vi "SequenceRunner.vi"() -> ()   [LabVIEW 2019]
uses:
  Components/B_Globals.vi
  Components/Global 2.vi
  Components/DeltaRamp_globals.vi
panel:
  in  "B_rate":dbl
  in  "T_rate":dbl
  out "Output File":path
  in  "Directory":path
  in  "T_high":dbl
  in  "T_low":dbl
  in  "Skip":bool
  out "Step":dbl
  out "Of":dbl
  out "Action":string="Waiting for go"
  in  "Start":bool
  in  "Array":T1(array[cluster])
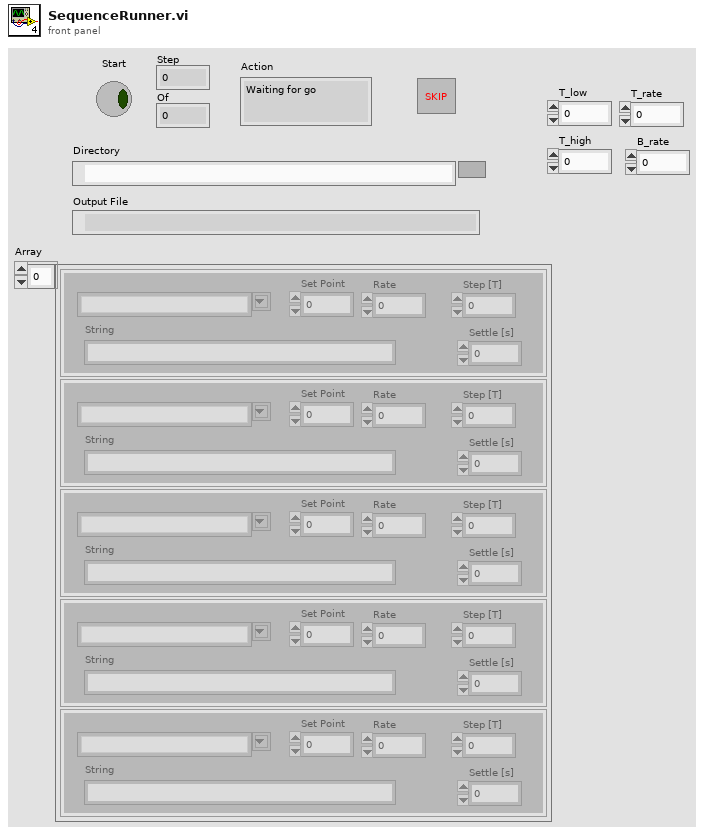
[diagram p1: front panel]
types:
  T1 = cluster{"Combo Box":string, "Rate":dbl, "Set Point":dbl, "String":string, "Step [T]":dbl, "Settle [s]":dbl}[]
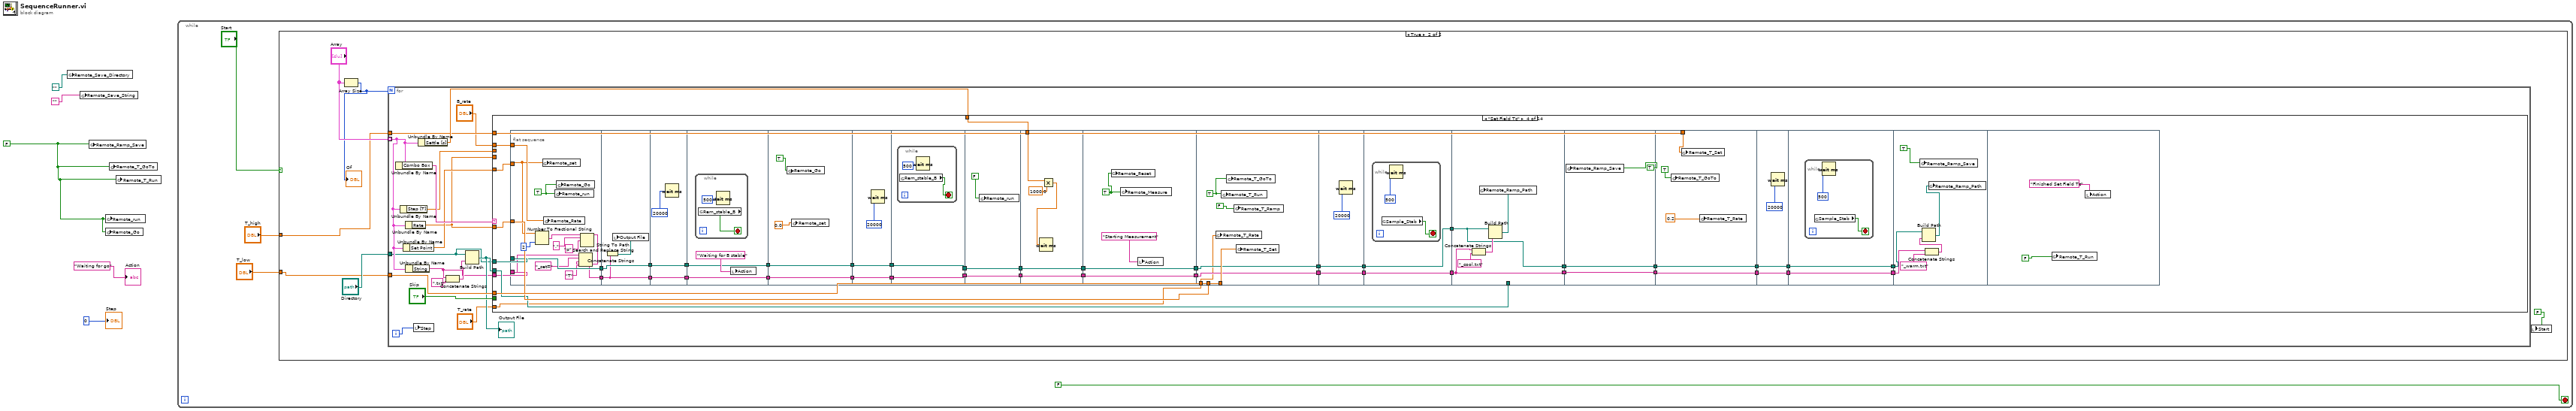
[diagram p0: block diagram]
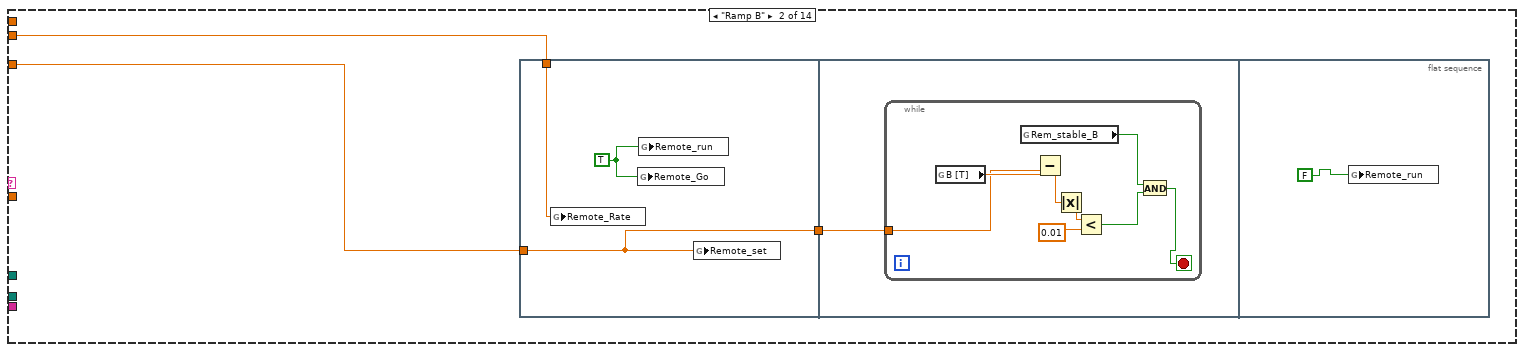
[diagram p4: hidden frame]
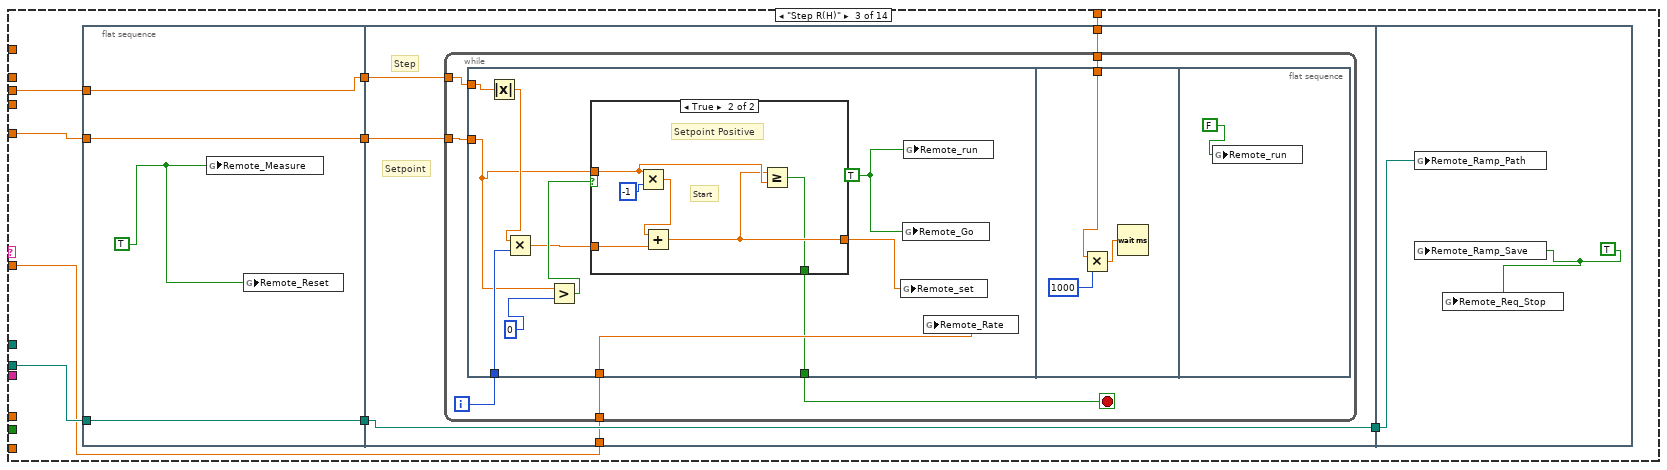
[diagram p5: hidden frame]
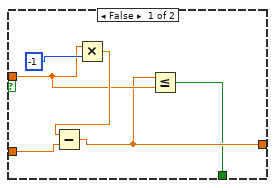
[diagram p6: hidden frame]
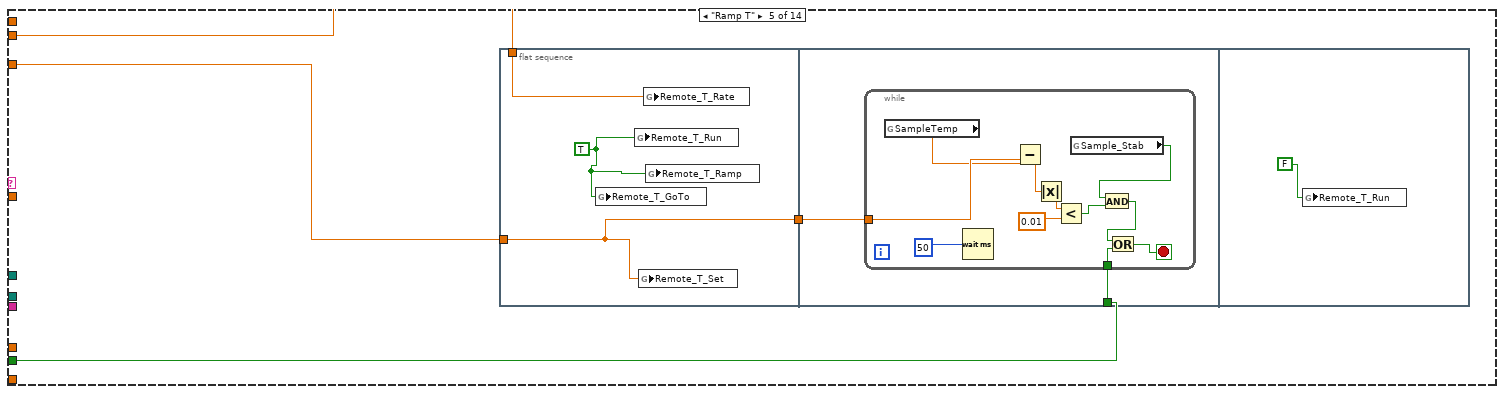
[diagram p7: hidden frame]
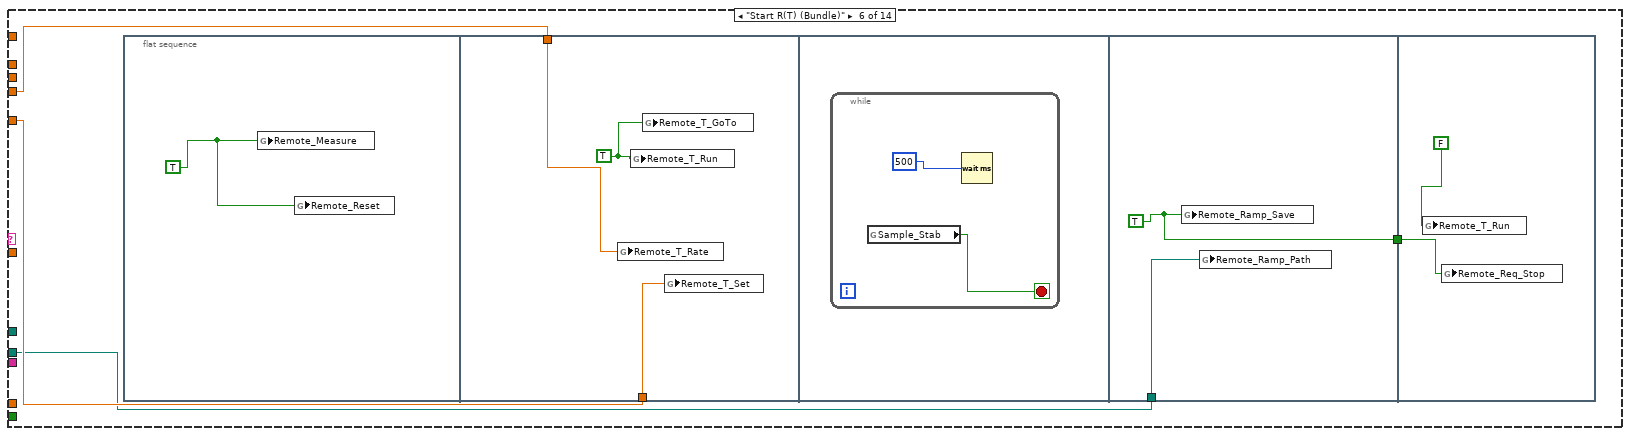
[diagram p8: hidden frame]
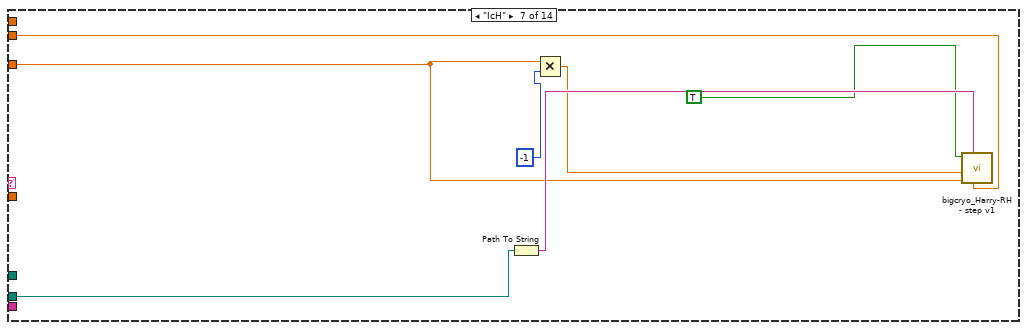
[diagram p9: hidden frame]
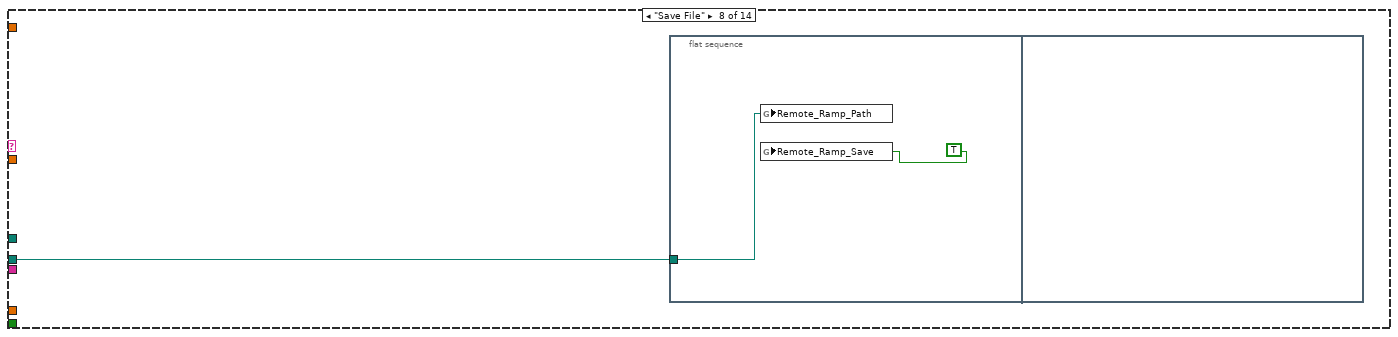
[diagram p10: hidden frame]
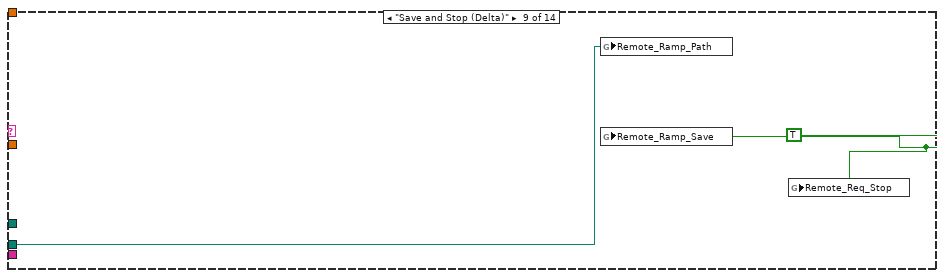
[diagram p11: hidden frame]
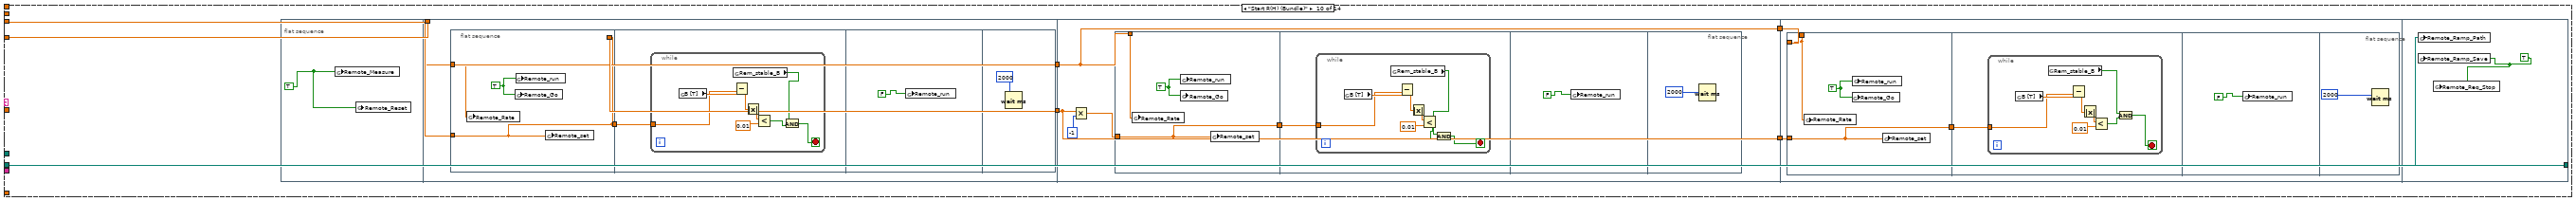
[diagram p12: hidden frame]
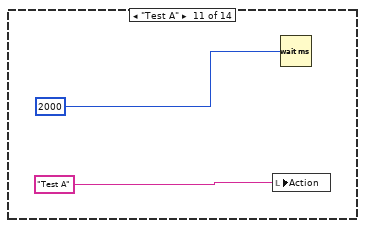
[diagram p13: hidden frame]
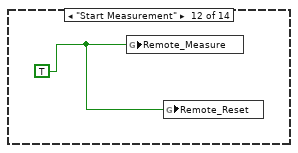
[diagram p14: hidden frame]
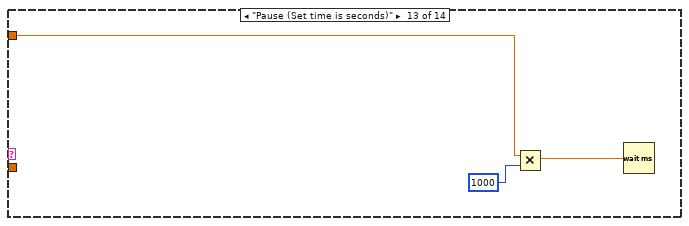
[diagram p15: hidden frame]
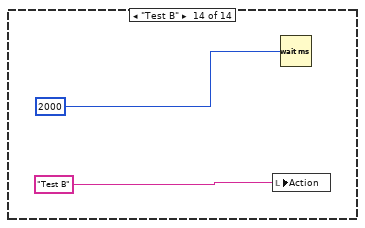
[diagram p16: hidden frame]
diagram:
  w5 = FALSE
  n1 = global write "DeltaRamp_globals.vi" "Remote_Save_Directory"(path "") -> ()
  n2 = global write "DeltaRamp_globals.vi" "Remote_Save_String"("") -> ()
  n3 = global write "DeltaRamp_globals.vi" "Remote_Ramp_Save"(w5) -> ()
  n4 = global write "B_Globals.vi" "Remote_Go"(w5) -> ()
  n5 = global write "B_Globals.vi" "Remote_run"(w5) -> ()
  n6 = global write "Global 2.vi" "Remote_T_GoTo"(w5) -> ()
  n7 = global write "Global 2.vi" "Remote_T_Run"(w5) -> ()
  n8 = while {
    stop <- FALSE stop-if-true
    n9 = case shown="True" "Start" {
      tunnel: "T_high" -> [_ w10]
      tunnel: "T_low" -> [_ w11]
      frame False {
      }
      frame True {
        n10 = Array Size(array="Array") -> (size(s)=w13:i32)
        "Of" <- w13
        n11 = for {
          N: w13 -> [_]
          tunnel: "Array" -> [w28] mode=indexing
          tunnel: "Directory" -> [w18]
          tunnel: w11 -> [w22]
          tunnel: w10 -> [w21]
          i -> [w30]
          n12 = Unbundle By Name(w28) -> ("Combo Box"=w32:string)
          n13 = Unbundle By Name(w28) -> ("Step [T]"=w26:dbl)
          n14 = Unbundle By Name(w28) -> ("Set Point"=w31:dbl)
          n15 = Unbundle By Name(w28) -> ("Rate"=w25:dbl)
          n16 = Unbundle By Name(w28) -> ("String"=w19:string)
          n17 = local write "Step"(w30) -> ()
          n18 = Unbundle By Name(w28) -> ("Settle [s]"=w27:dbl)
          n19 = Concatenate Strings(w19, ".txt") -> (w23:string)
          n20 = Build Path(base path=w18, name or relative path=w23) -> (appended path=w20:path)
          "Output File" <- w20
          n21 = case shown="\"Set Field Tc\"" w32 {
            tunnel: w31 -> [_ w35 w53 w147 w237 w260 w272 _ _ w289 _ _ w351 _]
            tunnel: w25 -> [_ w34 _ _ w238 w259 w277 _ _ w288 _ _ _ _]
            tunnel: w20 -> [_ _ w56 w142 _ w258 w274 w278 w282 w283 _ _ _ _]
            tunnel: "Skip" -> [_ _ _ _ w236 _ _ _ _ _ _ _ _ _]
            tunnel: w27 -> [_ _ w51 w146 _ _ _ _ _ _ _ _ _ _]
            tunnel: w26 -> [_ _ w50 _ _ _ _ _ _ _ _ _ _ _]
            tunnel: w25 -> [_ _ w49 w144 _ _ _ _ _ _ _ _ _ _]
            tunnel: w22 -> [_ _ _ w145 _ _ _ _ _ _ _ _ _ _]
            tunnel: w21 -> [_ _ _ w143 _ _ _ _ _ _ _ _ _ _]
            tunnel: w19 -> [_ _ _ w141 _ _ _ _ _ _ _ _ _ _]
            tunnel: w18 -> [_ _ _ w134 _ _ _ _ _ _ _ _ _ _]
            tunnel: "B_rate" -> [_ _ _ w111 _ _ _ _ _ _ _ _ _ _]
            tunnel: "T_rate" -> [_ _ _ w110 _ _ _ _ _ _ _ _ _ _]
            frame "False", Default {
            }
            frame "Ramp B" {
              n22 = flat-sequence {
                tunnel: w35 -> [w36]
                tunnel: w34 -> [w37]
                tunnel: [w36] -> w33
                tunnel: w33 -> [w39]
                frame #0 {
                  w38 = TRUE
                  n23 = global write "B_Globals.vi" "Remote_Rate"(w37) -> ()
                  n24 = global write "B_Globals.vi" "Remote_Go"(w38) -> ()
                  n25 = global write "B_Globals.vi" "Remote_run"(w38) -> ()
                  n26 = global write "B_Globals.vi" "Remote_set"(w36) -> ()
                }
                frame #1 {
                  n27 = while {
                    tunnel: w39 -> [w46]
                    stop <- w40 stop-if-true
                    n28 = global read "B_Globals.vi" "B [T]"() -> (w47:dbl)
                    n29 = global read "B_Globals.vi" "Rem_stable_B"() -> (w42:bool)
                    n30 = Subtract(x=w47, y=w46) -> (x-y=w45:dbl)
                    n31 = Absolute Value(x=w45) -> (abs(x)=w44:dbl)
                    n32 = Less?(x=w44, y=0.01) -> (x < y?=w41:bool)
                    n33 = And(x=w42, y=w41) -> (x .and. y?=w40:bool)
                  }
                }
                frame #2 {
                  n34 = global write "B_Globals.vi" "Remote_run"(FALSE) -> ()
                }
              }
            }
            frame "Step R(H)" {
              n35 = flat-sequence {
                tunnel: [w60] -> w57
                tunnel: w56 -> [w60]
                tunnel: [w59] -> w54
                tunnel: w53 -> [w59]
                tunnel: [w58] -> w52
                tunnel: w50 -> [w58]
                tunnel: w57 -> [w66]
                tunnel: [w66] -> w55
                tunnel: w54 -> [w65]
                tunnel: w52 -> [w64]
                tunnel: w51 -> [w63]
                tunnel: w49 -> [w62]
                tunnel: w55 -> [w100]
                frame #0 {
                  w61 = TRUE
                  n36 = global write "DeltaRamp_globals.vi" "Remote_Measure"(w61) -> ()
                  n37 = global write "DeltaRamp_globals.vi" "Remote_Reset"(w61) -> ()
                }
                frame #1 {
                  # "Step"
                  # "Setpoint"
                  n38 = while {
                    tunnel: w65 -> [w72]
                    tunnel: w64 -> [w70]
                    tunnel: w63 -> [w69]
                    tunnel: w62 -> [w68]
                    i -> [w71]
                    stop <- w67 stop-if-true
                    n39 = flat-sequence {
                      tunnel: w72 -> [w76]
                      tunnel: w71 -> [w82]
                      tunnel: w70 -> [w80]
                      tunnel: w68 -> [w79]
                      tunnel: [w73] -> w67
                      tunnel: w69 -> [w98]
                      frame #0 {
                        w81 = TRUE
                        n40 = Absolute Value(x=w80) -> (abs(x)=w83:dbl)
                        n41 = Multiply(x=w83, y=w82) -> (x*y=w75:dbl)
                        n42 = Greater?(x=w76, y=0) -> (0:w77:bool)
                        n43 = case shown="True" w77 {
                          tunnel: w76 -> [w86 w92]
                          tunnel: w75 -> [w88 w93]
                          tunnel: [w85 w91] -> w74
                          tunnel: [w84 w90] -> w73
                          frame False {
                            n44 = Multiply(x=w86, y=-1) -> (x*y=w87:dbl)
                            n45 = Subtract(x=w87, y=w88) -> (x-y=w85:dbl)
                            n46 = Less Or Equal?(x=w85, y=w86) -> (x <= y?=w84:bool)
                          }
                          frame True {
                            # "Start"
                            # "Setpoint Positive"
                            n47 = Multiply(x=w92, y=-1) -> (x*y=w94:dbl)
                            n48 = Add(x=w94, y=w93) -> (x+y=w91:dbl)
                            n49 = Greater Or Equal?(x=w91, y=w92) -> (x >= y?=w90:bool)
                          }
                        }
                        n50 = global write "B_Globals.vi" "Remote_set"(w74) -> ()
                        n51 = global write "B_Globals.vi" "Remote_Go"(w81) -> ()
                        n52 = global write "B_Globals.vi" "Remote_run"(w81) -> ()
                        n53 = global write "B_Globals.vi" "Remote_Rate"(w79) -> ()
                      }
                      frame #1 {
                        n54 = Multiply(x=w98, y=1000) -> (x*y=w97:dbl)
                        n55 = Wait (ms)(milliseconds to wait=w97) -> ()  [unwired: 1 out]
                      }
                      frame #2 {
                        n56 = global write "B_Globals.vi" "Remote_run"(FALSE) -> ()
                      }
                    }
                  }
                }
                frame #2 {
                  w101 = TRUE
                  n57 = global write "DeltaRamp_globals.vi" "Remote_Ramp_Path"(w100) -> ()
                  n58 = global write "DeltaRamp_globals.vi" "Remote_Ramp_Save"(w101) -> ()
                  n59 = global write "DeltaRamp_globals.vi" "Remote_Req_Stop"(w101) -> ()
                }
              }
            }
            frame "Set Field Tc" {
              n60 = flat-sequence {
                tunnel: w147 -> [w155]
                tunnel: w144 -> [_]
                tunnel: w111 -> [w159]
                tunnel: w141 -> [w157]
                tunnel: [w149] -> w136
                tunnel: [w158] -> w135
                tunnel: w134 -> [w158]
                tunnel: [w162] -> w105
                tunnel: w136 -> [w162]
                tunnel: w135 -> [w163]
                tunnel: [w163] -> w103
                tunnel: w105 -> [w166]
                tunnel: [w166] -> w104
                tunnel: w103 -> [w165]
                tunnel: [w165] -> w102
                tunnel: [w168] -> w137
                tunnel: w104 -> [w168]
                tunnel: [w167] -> w130
                tunnel: w102 -> [w167]
                tunnel: [w173] -> w138
                tunnel: w137 -> [w173]
                tunnel: [w172] -> w131
                tunnel: w130 -> [w172]
                tunnel: [w177] -> w139
                tunnel: w138 -> [w177]
                tunnel: [w176] -> w132
                tunnel: w131 -> [w176]
                tunnel: [w180] -> w140
                tunnel: w139 -> [w180]
                tunnel: [w179] -> w133
                tunnel: w132 -> [w179]
                tunnel: w140 -> [w183]
                tunnel: w133 -> [w184]
                tunnel: [w184] -> w127
                tunnel: [w183] -> w124
                tunnel: w146 -> [w189]
                tunnel: [w187] -> w128
                tunnel: w127 -> [w187]
                tunnel: [w186] -> w125
                tunnel: w124 -> [w186]
                tunnel: [w192] -> w129
                tunnel: w128 -> [w192]
                tunnel: [w191] -> w126
                tunnel: w125 -> [w191]
                tunnel: w145 -> [w199]
                tunnel: w144 -> [_]
                tunnel: w129 -> [w196]
                tunnel: w126 -> [w197]
                tunnel: [w197] -> w122
                tunnel: [w196] -> w120
                tunnel: w110 -> [w195]
                tunnel: [w202] -> w123
                tunnel: w122 -> [w202]
                tunnel: [w201] -> w121
                tunnel: w120 -> [w201]
                tunnel: w123 -> [w204]
                tunnel: w121 -> [w205]
                tunnel: [w205] -> w119
                tunnel: [w204] -> w118
                tunnel: w142 -> [_]
                tunnel: w119 -> [w210]
                tunnel: w118 -> [w209]
                tunnel: [w210] -> w109
                tunnel: [w209] -> w107
                tunnel: w109 -> [w215]
                tunnel: [w215] -> w108
                tunnel: w107 -> [w214]
                tunnel: [w214] -> w106
                tunnel: w143 -> [w220]
                tunnel: w108 -> [w216]
                tunnel: w106 -> [w217]
                tunnel: [w217] -> w115
                tunnel: [w216] -> w112
                tunnel: [w222] -> w117
                tunnel: w115 -> [w222]
                tunnel: [w221] -> w113
                tunnel: w112 -> [w221]
                tunnel: w117 -> [w225]
                tunnel: [w225] -> w116
                tunnel: [w224] -> w114
                tunnel: w113 -> [w224]
                tunnel: w116 -> [w231]
                tunnel: w114 -> [w230]
                frame #0 {
                  w160 = TRUE
                  n61 = Number To Fractional String(number=w155, precision (6)=2) -> (F-format string=w154:string)  [unwired: 2 in]
                  n62 = global write "B_Globals.vi" "Remote_set"(w155) -> ()
                  n63 = global write "B_Globals.vi" "Remote_Rate"(w159) -> ()
                  n64 = global write "B_Globals.vi" "Remote_run"(w160) -> ()
                  n65 = global write "B_Globals.vi" "Remote_Go"(w160) -> ()
                  n66 = Search and Replace String(input string=w154, search string=".", replace string="p") -> (result string=w151:string)  [unwired: 5 in, 3 out]
                  n67 = Concatenate Strings(w157, "_set=", w151, "T") -> (w149:string)
                }
                frame #1 {
                  n68 = String To Path(string=w162) -> (path=w161:path)
                  n69 = local write "Output File"(w161) -> ()
                }
                frame #2 {
                  n70 = Wait (ms)(milliseconds to wait=20000) -> ()  [unwired: 1 out]
                }
                frame #3 {
                  n71 = while {
                    stop <- w170 stop-if-true
                    n72 = global read "B_Globals.vi" "Rem_stable_B"() -> (w170:bool)
                    n73 = Wait (ms)(milliseconds to wait=500) -> ()  [unwired: 1 out]
                  }
                  n74 = local write "Action"("Waiting for B stable") -> ()
                }
                frame #4 {
                  n75 = global write "B_Globals.vi" "Remote_Go"(TRUE) -> ()
                  n76 = global write "B_Globals.vi" "Remote_set"(0.0) -> ()
                }
                frame #5 {
                  n77 = Wait (ms)(milliseconds to wait=20000) -> ()  [unwired: 1 out]
                }
                frame #6 {
                  n78 = while {
                    stop <- w182 stop-if-true
                    n79 = global read "B_Globals.vi" "Rem_stable_B"() -> (w182:bool)
                    n80 = Wait (ms)(milliseconds to wait=500) -> ()  [unwired: 1 out]
                  }
                }
                frame #7 {
                  n81 = global write "B_Globals.vi" "Remote_run"(FALSE) -> ()
                }
                frame #8 {
                  n82 = Multiply(x=w189, y=1000.0) -> (x*y=w188:dbl)
                  n83 = Wait (ms)(milliseconds to wait=w188) -> ()  [unwired: 1 out]
                }
                frame #9 {
                  w194 = TRUE
                  n84 = global write "DeltaRamp_globals.vi" "Remote_Reset"(w194) -> ()
                  n85 = global write "DeltaRamp_globals.vi" "Remote_Measure"(w194) -> ()
                  n86 = local write "Action"("Starting Measurement") -> ()
                }
                frame #10 {
                  w200 = TRUE
                  n87 = global write "Global 2.vi" "Remote_T_Rate"(w195) -> ()
                  n88 = global write "Global 2.vi" "Remote_T_Run"(w200) -> ()
                  n89 = global write "Global 2.vi" "Remote_T_GoTo"(w200) -> ()
                  n90 = global write "Global 2.vi" "Remote_T_Ramp"(FALSE) -> ()
                  n91 = global write "Global 2.vi" "Remote_T_Set"(w199) -> ()
                }
                frame #11 {
                  n92 = Wait (ms)(milliseconds to wait=20000) -> ()  [unwired: 1 out]
                }
                frame #12 {
                  n93 = while {
                    stop <- w207 stop-if-true
                    n94 = global read "Global 2.vi" "Sample_Stab"() -> (w207:bool)
                    n95 = Wait (ms)(milliseconds to wait=500) -> ()  [unwired: 1 out]
                  }
                }
                frame #13 {
                  n96 = Concatenate Strings(w209, "_cool.txt") -> (w211:string)
                  n97 = Build Path(base path=w210, name or relative path=w211) -> (appended path=w208:path)
                  n98 = global write "DeltaRamp_globals.vi" "Remote_Ramp_Path"(w208) -> ()
                }
                frame #14 {
                  n99 = global write "DeltaRamp_globals.vi" "Remote_Ramp_Save"(TRUE) -> ()
                }
                frame #15 {
                  n100 = global write "Global 2.vi" "Remote_T_GoTo"(TRUE) -> ()
                  n101 = global write "Global 2.vi" "Remote_T_Set"(w220) -> ()
                  n102 = global write "Global 2.vi" "Remote_T_Rate"(0.2) -> ()
                }
                frame #16 {
                  n103 = Wait (ms)(milliseconds to wait=20000) -> ()  [unwired: 1 out]
                }
                frame #17 {
                  n104 = while {
                    stop <- w227 stop-if-true
                    n105 = global read "Global 2.vi" "Sample_Stab"() -> (w227:bool)
                    n106 = Wait (ms)(milliseconds to wait=500) -> ()  [unwired: 1 out]
                  }
                }
                frame #18 {
                  n107 = global write "DeltaRamp_globals.vi" "Remote_Ramp_Save"(TRUE) -> ()
                  n108 = Concatenate Strings(w231, "_warm.txt") -> (w229:string)
                  n109 = Build Path(base path=w230, name or relative path=w229) -> (appended path=w228:path)
                  n110 = global write "DeltaRamp_globals.vi" "Remote_Ramp_Path"(w228) -> ()
                }
                frame #19 {
                  n111 = global write "Global 2.vi" "Remote_T_Run"(FALSE) -> ()
                  n112 = local write "Action"("Finished Set Field Tc") -> ()
                }
              }
            }
            frame "Ramp T" {
              n113 = flat-sequence {
                tunnel: w237 -> [w241]
                tunnel: [w241] -> w239
                tunnel: w238 -> [w242]
                tunnel: w239 -> [w244]
                tunnel: w236 -> [w243]
                frame #0 {
                  w240 = TRUE
                  n114 = global write "Global 2.vi" "Remote_T_GoTo"(w240) -> ()
                  n115 = global write "Global 2.vi" "Remote_T_Run"(w240) -> ()
                  n116 = global write "Global 2.vi" "Remote_T_Set"(w241) -> ()
                  n117 = global write "Global 2.vi" "Remote_T_Rate"(w242) -> ()
                  n118 = global write "Global 2.vi" "Remote_T_Ramp"(w240) -> ()
                }
                frame #1 {
                  n119 = while {
                    tunnel: w244 -> [w255]
                    tunnel: w243 -> [w249]
                    stop <- w250 stop-if-true
                    n120 = global read "Global 2.vi" "SampleTemp"() -> (w251:dbl)
                    n121 = Wait (ms)(milliseconds to wait=50) -> ()  [unwired: 1 out]
                    n122 = Subtract(x=w251, y=w255) -> (x-y=w254:dbl)
                    n123 = Absolute Value(x=w254) -> (abs(x)=w253:dbl)
                    n124 = Less?(x=w253, y=0.01) -> (x < y?=w247:bool)
                    n125 = global read "Global 2.vi" "Sample_Stab"() -> (w246:bool)
                    n126 = And(x=w246, y=w247) -> (x .and. y?=w245:bool)
                    n127 = Or(x=w245, y=w249) -> (x .or. y?=w250:bool)
                  }
                }
                frame #2 {
                  n128 = global write "Global 2.vi" "Remote_T_Run"(FALSE) -> ()
                }
              }
            }
            frame "Start R(T) (Bundle)" {
              n129 = flat-sequence {
                tunnel: w260 -> [w263]
                tunnel: w259 -> [w262]
                tunnel: w258 -> [w268]
                tunnel: [w267] -> w257
                tunnel: w257 -> [w269]
                frame #0 {
                  w261 = TRUE
                  n130 = global write "DeltaRamp_globals.vi" "Remote_Measure"(w261) -> ()
                  n131 = global write "DeltaRamp_globals.vi" "Remote_Reset"(w261) -> ()
                }
                frame #1 {
                  w264 = TRUE
                  n132 = global write "Global 2.vi" "Remote_T_Rate"(w262) -> ()
                  n133 = global write "Global 2.vi" "Remote_T_Run"(w264) -> ()
                  n134 = global write "Global 2.vi" "Remote_T_GoTo"(w264) -> ()
                  n135 = global write "Global 2.vi" "Remote_T_Set"(w263) -> ()
                }
                frame #2 {
                  n136 = while {
                    stop <- w265 stop-if-true
                    n137 = global read "Global 2.vi" "Sample_Stab"() -> (w265:bool)
                    n138 = Wait (ms)(milliseconds to wait=500) -> ()  [unwired: 1 out]
                  }
                }
                frame #3 {
                  w267 = TRUE
                  n139 = global write "DeltaRamp_globals.vi" "Remote_Ramp_Save"(w267) -> ()
                  n140 = global write "DeltaRamp_globals.vi" "Remote_Ramp_Path"(w268) -> ()
                }
                frame #4 {
                  n141 = global write "Global 2.vi" "Remote_T_Run"(FALSE) -> ()
                  n142 = global write "DeltaRamp_globals.vi" "Remote_Req_Stop"(w269) -> ()
                }
              }
            }
            frame "IcH" {
              n143 = Path To String(path=w274) -> (string=w275:string)
              n144 = Multiply(x=w272, y=-1) -> (x*y=w273:dbl)
              n145 = call "bigcryo_Harry-RH - step v1.vi"("Mag Field Step"=w277, "Directory Output"=w275, "Stop Field"=w272, "Start Field (T)"=w273, "Measure"=TRUE) -> ()  [unwired: 7 in]
            }
            frame "Save File" {
              n146 = flat-sequence {
                tunnel: w278 -> [w280]
                frame #0 {
                  n147 = global write "DeltaRamp_globals.vi" "Remote_Ramp_Path"(w280) -> ()
                  n148 = global write "DeltaRamp_globals.vi" "Remote_Ramp_Save"(TRUE) -> ()
                }
                frame #1 {
                }
              }
            }
            frame "Save and Stop (Delta)" {
              w281 = TRUE
              n149 = global write "DeltaRamp_globals.vi" "Remote_Ramp_Path"(w282) -> ()
              n150 = global write "DeltaRamp_globals.vi" "Remote_Ramp_Save"(w281) -> ()
              n151 = global write "DeltaRamp_globals.vi" "Remote_Req_Stop"(w281) -> ()
            }
            frame "Start R(H) (Bundle)" {
              n152 = flat-sequence {
                tunnel: w289 -> [w293]
                tunnel: w288 -> [w291]
                tunnel: [w292] -> w287
                tunnel: [w291] -> w286
                tunnel: w287 -> [w309]
                tunnel: w286 -> [w310]
                tunnel: [w310] -> w285
                tunnel: [w309] -> w284
                tunnel: w285 -> [w329]
                tunnel: w284 -> [w328]
                tunnel: w283 -> [w345]
                frame #0 {
                  w290 = TRUE
                  n153 = global write "DeltaRamp_globals.vi" "Remote_Measure"(w290) -> ()
                  n154 = global write "DeltaRamp_globals.vi" "Remote_Reset"(w290) -> ()
                }
                frame #1 {
                  n155 = flat-sequence {
                    tunnel: w293 -> [w295]
                    tunnel: [w295] -> w294
                    tunnel: w291 -> [w296]
                    tunnel: [w295] -> w292
                    tunnel: w294 -> [w298]
                    frame #0 {
                      w297 = TRUE
                      n156 = global write "B_Globals.vi" "Remote_Rate"(w296) -> ()
                      n157 = global write "B_Globals.vi" "Remote_Go"(w297) -> ()
                      n158 = global write "B_Globals.vi" "Remote_run"(w297) -> ()
                      n159 = global write "B_Globals.vi" "Remote_set"(w295) -> ()
                    }
                    frame #1 {
                      n160 = while {
                        tunnel: w298 -> [w305]
                        stop <- w299 stop-if-true
                        n161 = global read "B_Globals.vi" "B [T]"() -> (w306:dbl)
                        n162 = global read "B_Globals.vi" "Rem_stable_B"() -> (w300:bool)
                        n163 = Subtract(x=w306, y=w305) -> (x-y=w304:dbl)
                        n164 = Absolute Value(x=w304) -> (abs(x)=w303:dbl)
                        n165 = Less?(x=w303, y=0.01) -> (x < y?=w301:bool)
                        n166 = And(x=w300, y=w301) -> (x .and. y?=w299:bool)
                      }
                    }
                    frame #2 {
                      n167 = global write "B_Globals.vi" "Remote_run"(FALSE) -> ()
                    }
                    frame #3 {
                      n168 = Wait (ms)(milliseconds to wait=2000) -> ()  [unwired: 1 out]
                    }
                  }
                }
                frame #2 {
                  n169 = Multiply(x=w309, y=-1) -> (x*y=w311:dbl)
                  n170 = flat-sequence {
                    tunnel: w311 -> [w314]
                    tunnel: w310 -> [w315]
                    tunnel: [w314] -> w313
                    tunnel: w313 -> [w317]
                    frame #0 {
                      w316 = TRUE
                      n171 = global write "B_Globals.vi" "Remote_Rate"(w315) -> ()
                      n172 = global write "B_Globals.vi" "Remote_Go"(w316) -> ()
                      n173 = global write "B_Globals.vi" "Remote_run"(w316) -> ()
                      n174 = global write "B_Globals.vi" "Remote_set"(w314) -> ()
                    }
                    frame #1 {
                      n175 = while {
                        tunnel: w317 -> [w324]
                        stop <- w318 stop-if-true
                        n176 = global read "B_Globals.vi" "B [T]"() -> (w325:dbl)
                        n177 = global read "B_Globals.vi" "Rem_stable_B"() -> (w320:bool)
                        n178 = Subtract(x=w325, y=w324) -> (x-y=w323:dbl)
                        n179 = Absolute Value(x=w323) -> (abs(x)=w322:dbl)
                        n180 = Less?(x=w322, y=0.01) -> (x < y?=w319:bool)
                        n181 = And(x=w320, y=w319) -> (x .and. y?=w318:bool)
                      }
                    }
                    frame #2 {
                      n182 = global write "B_Globals.vi" "Remote_run"(FALSE) -> ()
                    }
                    frame #3 {
                      n183 = Wait (ms)(milliseconds to wait=2000) -> ()  [unwired: 1 out]
                    }
                  }
                }
                frame #3 {
                  n184 = flat-sequence {
                    tunnel: w328 -> [w332]
                    tunnel: [w331] -> _
                    tunnel: [w332] -> w330
                    tunnel: w329 -> [w331]
                    tunnel: w330 -> [w334]
                    frame #0 {
                      w333 = TRUE
                      n185 = global write "B_Globals.vi" "Remote_Rate"(w331) -> ()
                      n186 = global write "B_Globals.vi" "Remote_Go"(w333) -> ()
                      n187 = global write "B_Globals.vi" "Remote_run"(w333) -> ()
                      n188 = global write "B_Globals.vi" "Remote_set"(w332) -> ()
                    }
                    frame #1 {
                      n189 = while {
                        tunnel: w334 -> [w341]
                        stop <- w336 stop-if-true
                        n190 = global read "B_Globals.vi" "B [T]"() -> (w342:dbl)
                        n191 = global read "B_Globals.vi" "Rem_stable_B"() -> (w335:bool)
                        n192 = Subtract(x=w342, y=w341) -> (x-y=w340:dbl)
                        n193 = Absolute Value(x=w340) -> (abs(x)=w339:dbl)
                        n194 = Less?(x=w339, y=0.01) -> (x < y?=w337:bool)
                        n195 = And(x=w335, y=w337) -> (x .and. y?=w336:bool)
                      }
                    }
                    frame #2 {
                      n196 = global write "B_Globals.vi" "Remote_run"(FALSE) -> ()
                    }
                    frame #3 {
                      n197 = Wait (ms)(milliseconds to wait=2000) -> ()  [unwired: 1 out]
                    }
                  }
                }
                frame #4 {
                  w346 = TRUE
                  n198 = global write "DeltaRamp_globals.vi" "Remote_Ramp_Path"(w345) -> ()
                  n199 = global write "DeltaRamp_globals.vi" "Remote_Ramp_Save"(w346) -> ()
                  n200 = global write "DeltaRamp_globals.vi" "Remote_Req_Stop"(w346) -> ()
                }
              }
            }
            frame "Test A" {
              n201 = local write "Action"("Test A") -> ()
              n202 = Wait (ms)(milliseconds to wait=2000) -> ()  [unwired: 1 out]
            }
            frame "Start Measurement" {
              w349 = TRUE
              n203 = global write "DeltaRamp_globals.vi" "Remote_Measure"(w349) -> ()
              n204 = global write "DeltaRamp_globals.vi" "Remote_Reset"(w349) -> ()
            }
            frame "Pause (Set time is seconds)" {
              n205 = Multiply(x=w351, y=1000) -> (x*y=w350:dbl)
              n206 = Wait (ms)(milliseconds to wait=w350) -> ()  [unwired: 1 out]
            }
            frame "Test B" {
              n207 = local write "Action"("Test B") -> ()
              n208 = Wait (ms)(milliseconds to wait=2000) -> ()  [unwired: 1 out]
            }
          }
        }
        n209 = local write "Start"(FALSE) -> ()
      }
    }
  }
  "Action" <- "Waiting for go"
  "Step" <- 0
